vi "Material.Build Palette Array.vi"(10 "palette":T1={"0"="0", "5"="0", "10"="0", "15"="0", "20"="0", "25"="0", "30"="0", "35"="0", "40"="0", "50"="0", "60"="0", "70"="0", "80"="0", "90"="0", "95"="0", "98"="0", "99"="0", "100"="0"}, 11 "Name":string) -> (2 "Palettes":refnum<class "Material-Palette.lvclass">)   [LabVIEW 2021, in "TSC Material Theme.lvlib" / "Material-Palette.lvclass"]
doc: "Convert the json represenation of the palette colors into array of class palettes.\n\n<b>Code Developed By:</b>\nTechnology Service Corporation\nwww.tsc.com/atcs\n\nDeveloper:\nDaniel Coons"
uses:
  Material-Palette.lvclass
  Material-Palette.lvclass/Material-Palette.ctl
  TSC Material Theme.lvlib
  _Material Theme SubVIs/material json palette.ctl
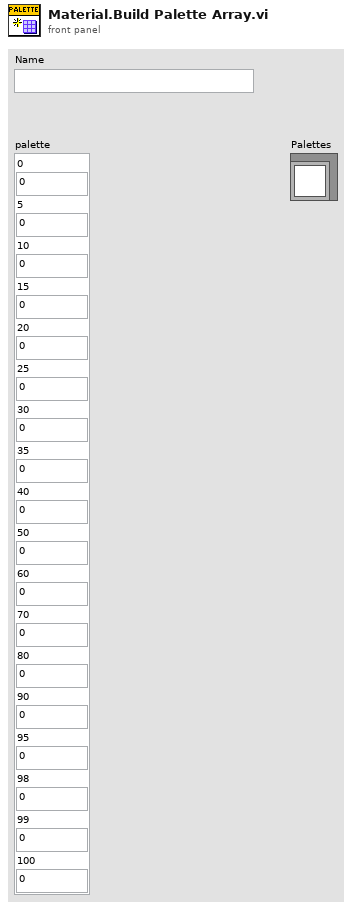
[diagram p1: front panel]
types:
  T1 = typedef "material json palette.ctl" = cluster{"0":string, "5":string, "10":string, "15":string, "20":string, "25":string, "30":string, "35":string, "40":string, "50":string, "60":string, "70":string, "80":string, "90":string, "95":string, "98":string, "99":string, "100":string}
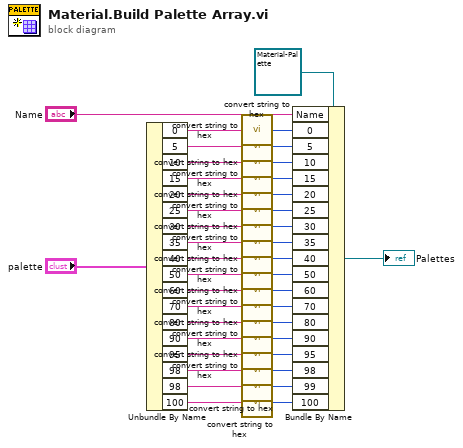
[diagram p0: block diagram]
diagram:
  n1 = Unbundle By Name("palette") -> ("0"=w38:string, "5"=w37:string, "10"=w36:string, "15"=w35:string, "20"=w34:string, "25"=w33:string, "30"=w32:string, "35"=w31:string, "40"=w30:string, "50"=w29:string, "60"=w28:string, "70"=w27:string, "80"=w26:string, "90"=w25:string, "95"=w24:string, "98"=w23:string, "98"=w22:string, "100"=w21:string)
  n2 = call "convert string to hex.vi"("string"=w38) -> ("hex"=w19:u32)
  n3 = call "convert string to hex.vi"("string"=w37) -> ("hex"=w2:u32)
  n4 = call "convert string to hex.vi"("string"=w36) -> ("hex"=w3:u32)
  n5 = call "convert string to hex.vi"("string"=w35) -> ("hex"=w4:u32)
  n6 = call "convert string to hex.vi"("string"=w34) -> ("hex"=w5:u32)
  n7 = call "convert string to hex.vi"("string"=w33) -> ("hex"=w6:u32)
  n8 = call "convert string to hex.vi"("string"=w32) -> ("hex"=w7:u32)
  n9 = call "convert string to hex.vi"("string"=w31) -> ("hex"=w8:u32)
  n10 = call "convert string to hex.vi"("string"=w30) -> ("hex"=w9:u32)
  n11 = call "convert string to hex.vi"("string"=w29) -> ("hex"=w10:u32)
  n12 = call "convert string to hex.vi"("string"=w28) -> ("hex"=w11:u32)
  n13 = call "convert string to hex.vi"("string"=w27) -> ("hex"=w12:u32)
  n14 = call "convert string to hex.vi"("string"=w26) -> ("hex"=w13:u32)
  n15 = call "convert string to hex.vi"("string"=w25) -> ("hex"=w14:u32)
  n16 = call "convert string to hex.vi"("string"=w24) -> ("hex"=w15:u32)
  n17 = call "convert string to hex.vi"("string"=w23) -> ("hex"=w16:u32)
  n18 = call "convert string to hex.vi"("string"=w22) -> ("hex"=w17:u32)
  n19 = call "convert string to hex.vi"("string"=w21) -> ("hex"=w18:u32)
  n20 = Bundle By Name(cluster=refnum<class "Material-Palette.lvclass"> refnum ("Material-Palette.lvclass"), "Name"="Name", "0"=w19, "5"=w2, "10"=w3, "15"=w4, "20"=w5, "25"=w6, "30"=w7, "35"=w8, "40"=w9, "50"=w10, "60"=w11, "70"=w12, "80"=w13, "90"=w14, "95"=w15, "98"=w16, "99"=w17, "100"=w18) -> (→"Palettes":refnum<class "Material-Palette.lvclass">)
